vi "Simu_sinus_Pid.vi"() -> ()   [LabVIEW 2026]
uses:
  <vilib>/addons/control/pid/pid.llb/PID (DBL).vi
  <vilib>/addons/control/pid/NI_PID_pid.lvlib
panel:
  in  "n millisecondes":u32
  in  "stop":bool
  in  "Switch":bool
  in  "reinitialize? (F)":bool caption="réinitialiser ? (F)"
  in  "dt (s)":dbl=-1.0 format="%#_13g"
  in  "Tension Max":dbl=100.0
  in  "Plage de pixel":dbl=200.0
  in  "nbr de pixels":dbl=100.0
  in  "PID gains":T1={"proportional gain (Kc)"=0.95, "integral time (Ti, min)"=0.001, "derivative time (Td, min)"=0.0} caption="gains du PID" {"derivative time (Td, min)" format="%.3f"; "integral time (Ti, min)" format="%.3f"; "proportional gain (Kc)" format="%.3f"}
  out "PID":dbl(graph)=0.36903498472722396
  out "output":dbl=0.36903498472722396
  in  "output range":cluster{"output high":dbl, "output low":dbl}={"output high"=100.0, "output low"=0.0} caption="gamme de la sortie" {"output low" format="%.2f"; "output high" format="%.2f"}
  out "Signal/correction":cluster{dbl, dbl}(graph)
  in  "Ech":i32=2000
  in  "Fréquence":dbl=100.0
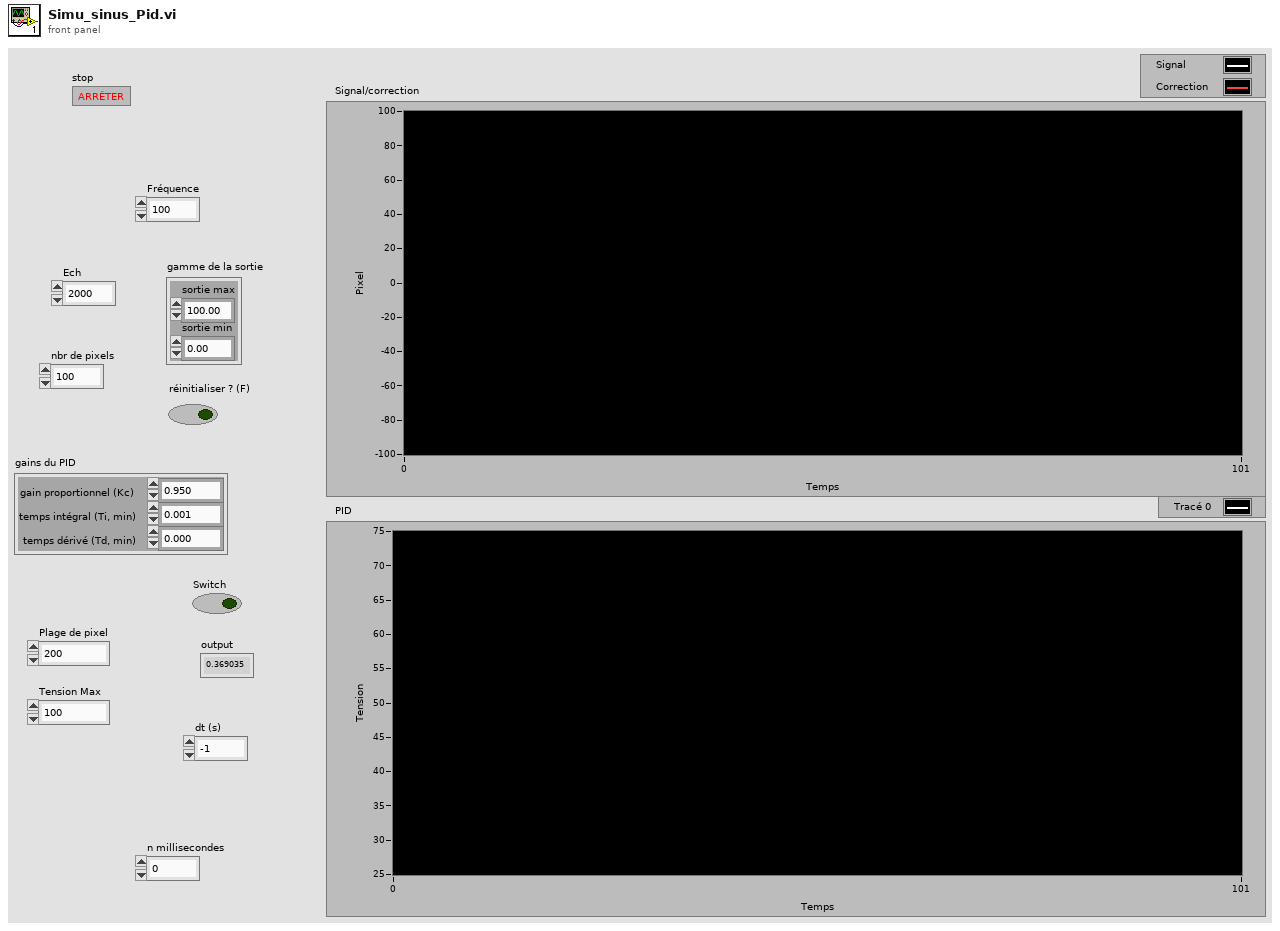
[diagram p1: front panel]
types:
  T1 = cluster{"proportional gain (Kc)":dbl, "integral time (Ti, min)":dbl, "derivative time (Td, min)":dbl}
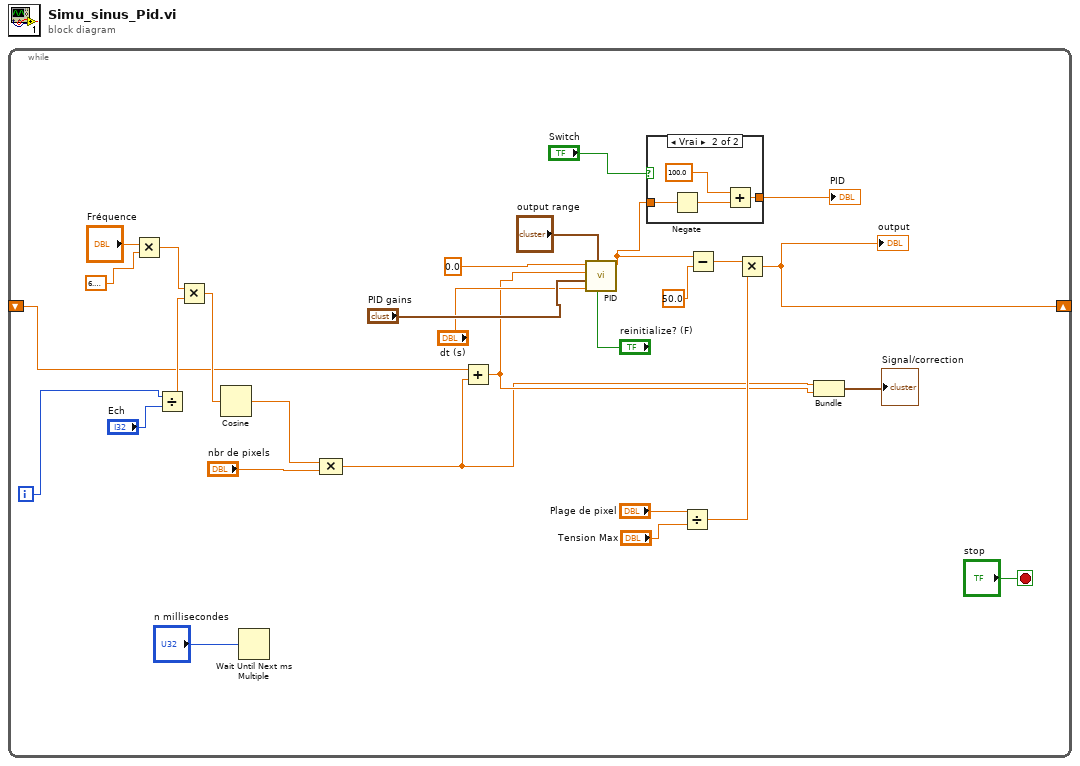
[diagram p0: block diagram]
diagram:
  n1 = while {
    shift-right: [w13] -> _
    shift-left: _ -> [w21]
    i -> [w27]
    stop <- "stop" stop-if-true
    n2 = Multiply(x="Fréquence", y=6.283185307179586) -> (x*y=w25:dbl)
    n3 = Divide(x=w27, y="Ech") -> (x/y=w24:dbl)
    n4 = Multiply(x=w25, y=w24) -> (x*y=w23:dbl)
    n5 = Cosine(x=w23) -> (cos(x)=w18:dbl)
    n6 = Wait Until Next ms Multiple(millisecond multiple="n millisecondes") -> ()  [unwired: 1 out]
    n7 = Compound Arithmetic op=MULTIPLY(w18, "nbr de pixels") -> (w3:dbl)
    n8 = Add(x=w21, y=w3) -> (x+y=w8:dbl)
    n9 = call-poly <vilib>:"PID.vi"("reinitialize? (F)"="reinitialize? (F)", "output range"="output range", "dt (s)"="dt (s)", "PID gains"="PID gains", "process variable"=w8, "setpoint"=0.0) -> ("output"=w16:dbl)  [unwired: 4 in, 1 out]
    n10 = case shown="Vrai" "Switch" {
      tunnel: w16 -> [w30 w34]
      tunnel: [w30 w32] -> w5
      frame False {
      }
      frame True {
        n11 = Negate(x=w34) -> (-x=w33:dbl)
        n12 = Add(x=100.0, y=w33) -> (x+y=w32:dbl)
      }
    }
    "PID" <- w5
    n13 = Divide(x="Plage de pixel", y="Tension Max") -> (x/y=w10:dbl)
    n14 = Subtract(x=w16, y=50.0) -> (x-y=w14:dbl)
    n15 = Multiply(x=w14, y=w10) -> (x*y=w13:dbl)
    "output" <- w13
    n16 = Bundle(w3, w8) -> (→"Signal/correction":cluster{dbl, dbl})  [unwired: 1 in]
  }
